vi "GetDigitizerBdcstEvents.vi"() -> (3 "Event Registration Refnum":refnum<event-registration>)   [LabVIEW 2014, in "Test.lvclass"]
uses:
  Test.lvclass
  Digitizer/DigitizerModule/Protected/clEventType.ctl
  Digitizer/DigitizerModule/DigitizerModule.lvlib
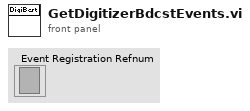
[diagram p1: front panel]
types:
  T1 = typedef "DigitizerModule.lvlib/clBroadcastEvents.ctl" = cluster{"DidInit":refnum<user-event>, "StatusUpdate":refnum<user-event>, "ErrorReport":refnum<user-event>, "DidStop":refnum<user-event>, "PathToINI":refnum<user-event>, "Channels":refnum<user-event>, "Acq":refnum<user-event>, "Trigger":refnum<user-event>, "Waveforms":refnum<user-event>}
  T2 = cluster{"Channels":refnum<user-event>, "Acq":refnum<user-event>, "Trigger":refnum<user-event>, "Waveforms":refnum<user-event>, "ErrorReport":refnum<user-event>}
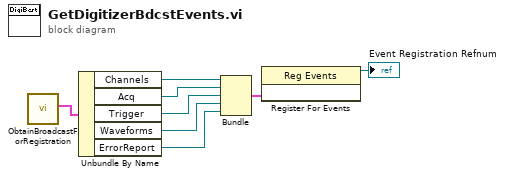
[diagram p0: block diagram]
diagram:
  n1 = call "ObtainBroadcastForRegistration.vi"() -> ("clDigitizerBdcstEvents"=w8:T1)  [unwired: 10 in, 1 out]
  n2 = Unbundle By Name(w8) -> ("Channels"=w7:refnum<user-event>, "Acq"=w6:refnum<user-event>, "Trigger"=w4:refnum<user-event>, "Waveforms"=w3:refnum<user-event>, "ErrorReport"=w2:refnum<user-event>)
  n3 = Bundle("Channels"=w7, "Acq"=w6, "Trigger"=w4, "Waveforms"=w3, "ErrorReport"=w2) -> (w5:T2)  [unwired: 1 in]
  n4 = register-events(w5) -> (reference out=→"Event Registration Refnum":refnum<event-registration>)  [unwired: 2 in, 1 out]
